vi "recover module.vi"(11 "recovery request":T1) -> (3 "response":T2)   [LabVIEW 2013, in "worker pool.lvlib"]
uses:
  worker pool.lvlib
  recovery response.ctl
  <vilib>/NI/Tag Bus Module Framework/runtime/TBM module execution interface.lvclass
  recovery request.ctl
  <vilib>/NI/Tag Bus Module Framework/module configuration/TBM module configuration.lvclass
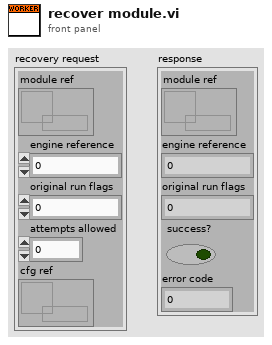
[diagram p1: front panel]
types:
  T1 = typedef "worker pool.lvlib/recovery request.ctl" = cluster{"module ref":refnum<data-value>, "engine reference":i32, "original run flags":u8, "attempts allowed":u16, "cfg ref":refnum<data-value>}
  T2 = typedef "worker pool.lvlib/recovery response.ctl" = cluster{"module ref":refnum<data-value>, "engine reference":i32, "original run flags":u8, "success?":bool, "error code":i32}
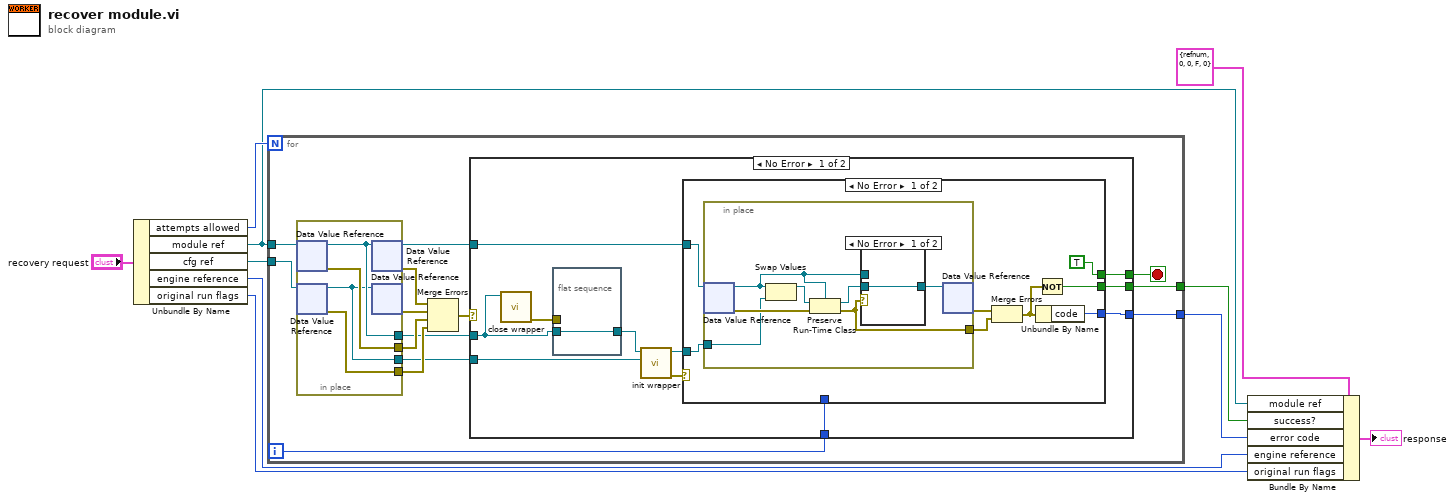
[diagram p0: block diagram]
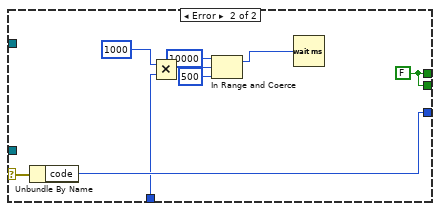
[diagram p3: hidden frame]
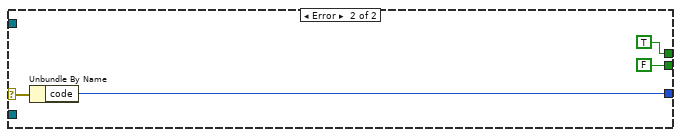
[diagram p4: hidden frame]
diagram:
  n1 = Unbundle By Name("recovery request") -> ("attempts allowed"=w7:u16, "module ref"=w1:refnum<data-value>, "cfg ref"=w4:refnum<data-value>, "engine reference"=w6:i32, "original run flags"=w5:u8)
  n2 = for {
    N: w7 -> [_]
    tunnel: w4 -> [w24]
    tunnel: w1 -> [w23]
    tunnel: [w18] -> w3
    tunnel: [w16] -> w2
    i -> [w11]
    stop <- w15 stop-if-true
    n3 = in-place {
      in-place-border: [w70] -> w20
      in-place-border: [w69] -> w19
      in-place-border: [w68] -> w14
      in-place-border: [w67] -> w13
      n4 = in-place-dvr #1(w23) -> (w68:refnum<class "TBM module execution interface.lvclass">, w70:errorcluster)
      n5 = in-place-dvr #2(w24) -> (w67:refnum<class "TBM module configuration.lvclass">, w69:errorcluster)
      n6 = in-place-dvr #1(w68) -> (w12:refnum<data-value>, w22:errorcluster)
      n7 = in-place-dvr #2(w67) -> (w21:errorcluster)  [unwired: 1 out]
    }
    n8 = Merge Errors(w22, w21, w20, w19) -> (w17:errorcluster)
    n9 = case shown="No Error" w17 {
      selector: w17 -> [_ w65]
      tunnel: [w28 FALSE] -> w18
      tunnel: [w30 w64] -> w16
      tunnel: [w29 TRUE] -> w15
      tunnel: w14 -> [w33 _]
      tunnel: w13 -> [w32 _]
      tunnel: w12 -> [w27 _]
      tunnel: w11 -> [w25 _]
      frame No Error {
        n10 = call <vilib>:"close wrapper.vi"("module in"=w33) -> ("error out"=w35:errorcluster)  [unwired: 10 in]
        n11 = flat-sequence {
          tunnel: w35 -> [_]
          tunnel: [w62] -> w34
          tunnel: w33 -> [w62]
          frame #0 {
          }
        }
        n12 = call <vilib>:"init wrapper.vi"("module configuration"=w32, "module in"=w34) -> ("error out"=w31:errorcluster, "module out"=w26:refnum<class "TBM module execution interface.lvclass">)  [unwired: 6 in, 2 out]
        n13 = case shown="No Error" w31 {
          selector: w31 -> [_ w61]
          tunnel: [w37 w60] -> w30
          tunnel: [TRUE w59] -> w29
          tunnel: [w40 w59] -> w28
          tunnel: w27 -> [w43 _]
          tunnel: w26 -> [w36 _]
          tunnel: w25 -> [_ w57]
          frame No Error {
            n14 = in-place {
              in-place-border: [w47] -> w41
              in-place-border: w36 -> [w49]
              n15 = in-place-dvr #3(w43) -> (w44:refnum<class "TBM module execution interface.lvclass">, w50:errorcluster)
              n16 = Swap Values(12:w44, 14:w49) -> (1:w48:refnum<class "TBM module execution interface.lvclass">)  [unwired: 1 in, 1 out]
              n17 = Preserve Run-Time Class(object in=w48, error in=w50, 2:w44) -> (object out=w45:refnum<class "TBM module execution interface.lvclass">, error out=w47:errorcluster)
              n18 = case shown="No Error" w47 {
                tunnel: [w51 w52] -> w46
                tunnel: w45 -> [w51 _]
                tunnel: w44 -> [_ w52]
                frame No Error {
                }
                frame Error {
                }
              }
              n19 = in-place-dvr #3(w46) -> (w42:errorcluster)  [unwired: 1 out]
            }
            n20 = Merge Errors(w42, w41) -> (w38:errorcluster)
            n21 = Unbundle By Name(w38) -> ("code"=w37:i32)
            n22 = Not(x=w38) -> (.not. x?=w40:bool)
          }
          frame Error {
            w59 = FALSE
            n23 = Unbundle By Name(w61) -> ("code"=w60:i32)
            n24 = Multiply(x=u32 1000 ("milliseconds to wait"), y=w57) -> (x*y=w56:u32)
            n25 = In Range and Coerce(upper limit=u32 10000, x=w56, lower limit=u32 500) -> (coerced(x)=w54:u32)  [unwired: 1 out]
            n26 = Wait (ms)(milliseconds to wait=w54) -> ()  [unwired: 1 out]
          }
        }
      }
      frame Error {
        n27 = Unbundle By Name(w65) -> ("code"=w64:i32)
      }
    }
  }
  n28 = Bundle By Name(cluster=T2 {"module ref"=refnum, "engine reference"=0, "original run flags"=0, "success?"=FALSE, "error code"=0} ("element"), "module ref"=w1, "success?"=w3, "error code"=w2, "engine reference"=w6, "original run flags"=w5) -> (→"response":T2)
